vi "Initialize Routing Channels Page.vi"(8 "error in (no error)":errorcluster, 10 "Main Page Controls":T2, 11 "Item Ref in":T1 format="%.0x") -> (0 "error out":errorcluster, 3 "Item Ref out":T1 format="%.0x")   [LabVIEW 2017, in "Routing and Faulting System Explorer.lvlib"]
uses:
  Routing and Faulting System Explorer.lvlib
  Main Page Controls.ctl
  <vilib>/NI Veristand/Custom Device API/Custom Device Item Ref.ctl
  <vilib>/NI VeriStand/Custom Device API/Custom Device API.lvlib
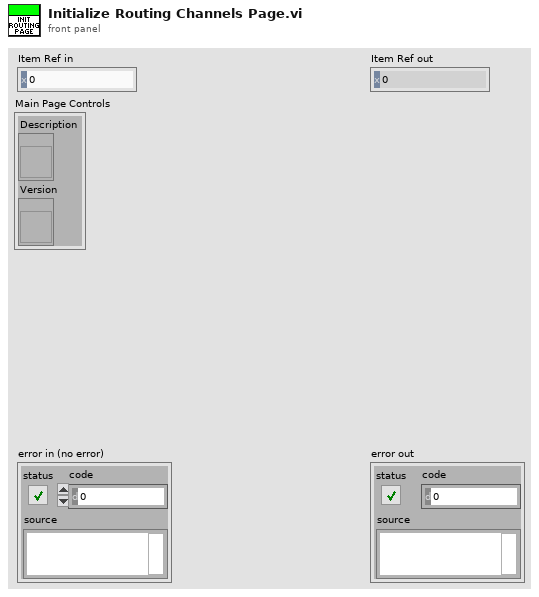
[diagram p1: front panel]
types:
  T1 = typedef "Custom Device API.lvlib/Custom Device Item Ref.ctl" = u64
  T2 = typedef "Routing and Faulting System Explorer.lvlib/Main Page Controls.ctl" = cluster{"Description":refnum<vi>, "Version":refnum<vi>}
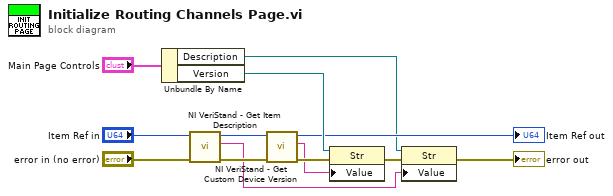
[diagram p0: block diagram]
diagram:
  n1 = Unbundle By Name("Main Page Controls") -> ("Description"=w1:refnum<vi>, "Version"=w10:refnum<vi>)
  n2 = call <vilib>:"NI VeriStand - Get Item Description.vi"("error in (no error)"="error in (no error)", "Item Ref in"="Item Ref in") -> ("error out"=w4:errorcluster, "Description"=w2:string, "Item Ref out"=w5:T1)  [unwired: 6 in, 1 out]
  n3 = call <vilib>:"NI VeriStand - Get Custom Device Version.vi"("error in (no error)"=w4, "Device Ref in"=w5) -> ("error out"=w9:errorcluster, "Value"=w3:string, "Device Ref out"=→"Item Ref out":T1)  [unwired: 7 in]
  n4 = property class="Str"(reference=w10, error in=w9, "Value"=w3) -> (error out=w11:errorcluster)  [unwired: 1 out]
  n5 = property class="Str"(reference=w1, error in=w11, "Value"=w2) -> (error out=→"error out":errorcluster)  [unwired: 1 out]
